vi "CollectImageSet (SubVI).vi"(0 "Session in":T1, 1 "Path to save collected images":path=path "E:/XYZstage+Camera_CollectedImages/12-17-2016/images", 3 "Stage position":refnum<vi>, 5 "Set of Coordinates to Process":dbl[][](array[numeric]), 8 "Current image":refnum<vi>, 9 "Axes Speeds [mm/s]":T4={"X Speed"=10.0, "Y Speed"=10.0, "Z Speed"=10.0}, 11 "error in":errorcluster, 13 "Moving":refnum<vi>) -> (4 "Session out":T1, 6 "Captured positions":dbl[][](array[numeric]), 10 "Image Array":T2[](array[plugin-control])=["remote image 0000000013A07714", "remote image 0000000013A076AC", "remote image 0000000013A0777C", "remote image 0000000013A077E4", "remote image 0000000013A0784C", "image_5", "image_6", "image_7", "image_8", "image_9", "image_10", "image_11", "image_12", "image_13", "image_14", "image_15", "image_16", "image_17", "image_18", "image_19", "image_20", "image_21", "image_22", "image_23", "image_24", "image_25", "image_26", "image_27", "image_28", "image_29", "image_30", "image_31", "image_32", "image_33", "image_34", "image_35", "image_36", "image_37", "image_38", "image_39", "image_40", "image_41", "image_42", "image_43", "image_44", "image_45", "image_46", "image_47", "image_48", "image_49", "image_50", "image_51", "image_52", "image_53", "image_54", "image_55", "image_56", "image_57", "image_58", "image_59", "image_60", "image_61", "image_62", "image_63", "image_64", "image_65", "image_66", "image_67", "image_68", "image_69", "image_70", "image_71", "image_72", "image_73", "image_74", "image_75", "image_76", "image_77", "image_78", "image_79"], 14 "Finished!":bool, 15 "error out":errorcluster)   [LabVIEW 2016]
uses:
  <vilib>/userdefined/High Color/IMAQdx.ctl
  <vilib>/vision/driver/NI_Vision_Acquisition_Software.lvlib
  <vilib>/vision/NI_Vision_Development_Module.lvlib
panel:
  out "Most recently collected image":T2(plugin-control)
  out "Image #":i32
  out "XYZ Stage Current Position":T3
  out "Moving":bool
  out "Object Location [mm]":T5
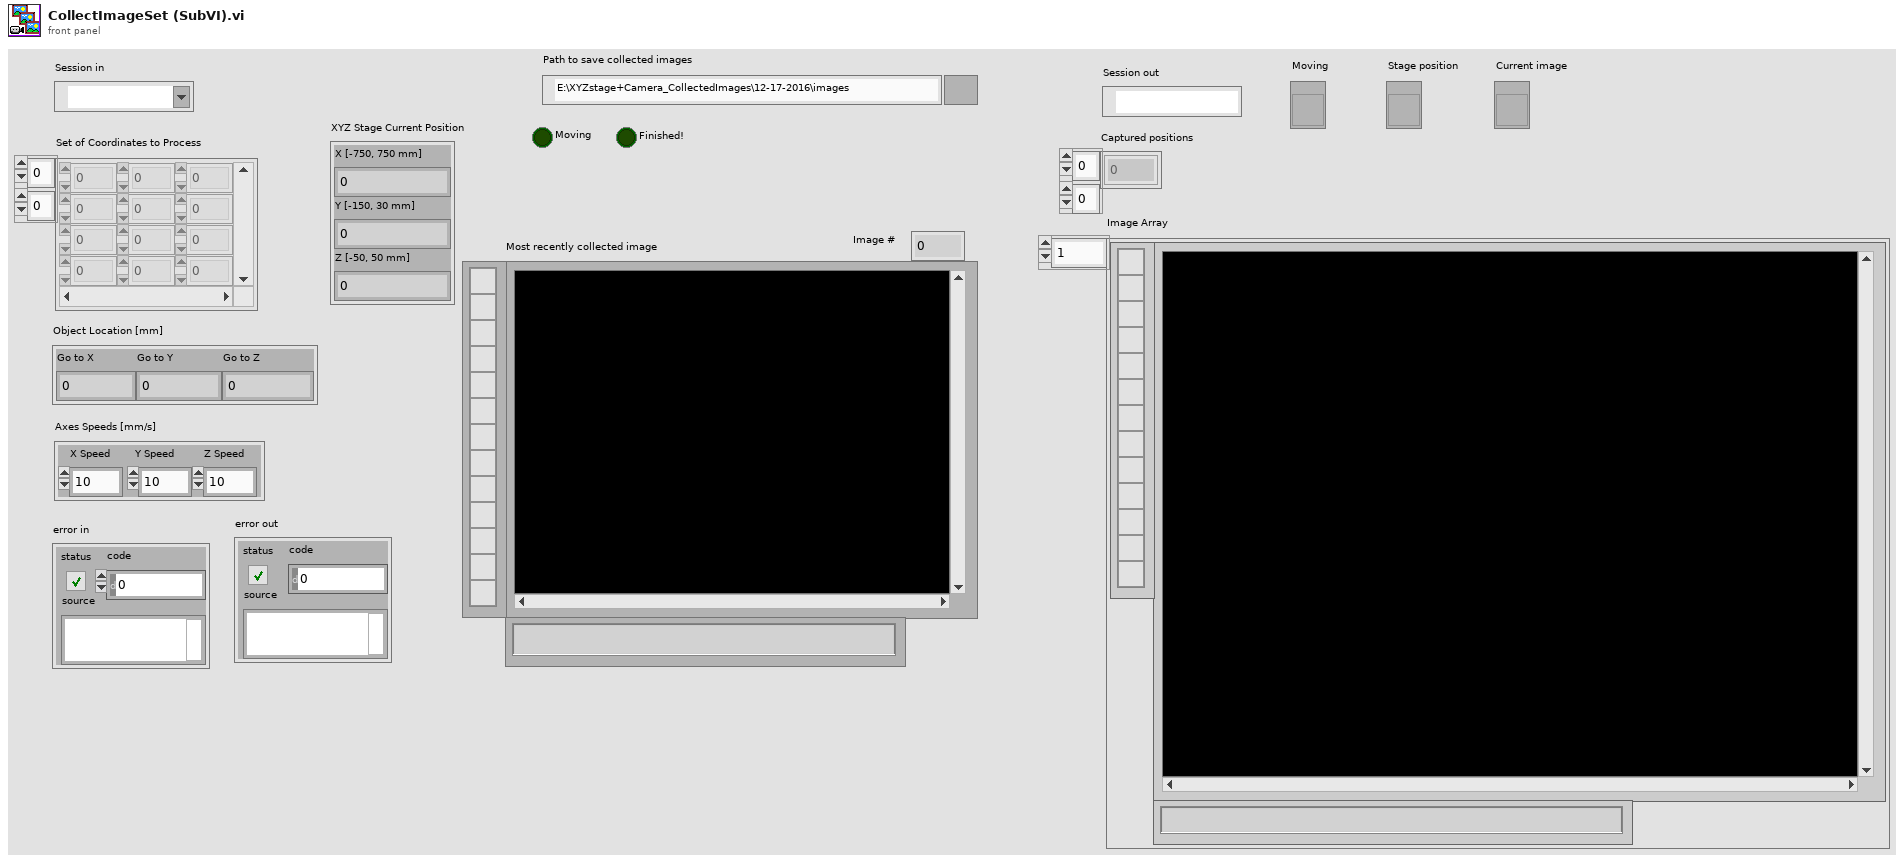
[diagram p1: front panel]
types:
  T1 = typedef "IMAQdx.ctl" = refnum<k21>
  T2 = typedef "IMAQ Image.ctl" = refnum<image>
  T3 = cluster{"X [-750, 750 mm]":dbl, "Y [-150, 30 mm]":dbl, "Z [-50, 50 mm]":dbl}
  T4 = cluster{"X Speed":dbl, "Y Speed":dbl, "Z Speed":dbl}
  T5 = cluster{"Go to X":dbl, "Go to Y":dbl, "Go to Z":dbl}
  T6 = cluster{"Set of Coordinates to Process[0]":dbl, "Set of Coordinates to Process[1]":dbl, "Set of Coordinates to Process[2]":dbl}
  T7 = typedef "Image Type" = u32
  T8 = cluster{"Final X":dbl, "Final Y":dbl, "Final Z":dbl}
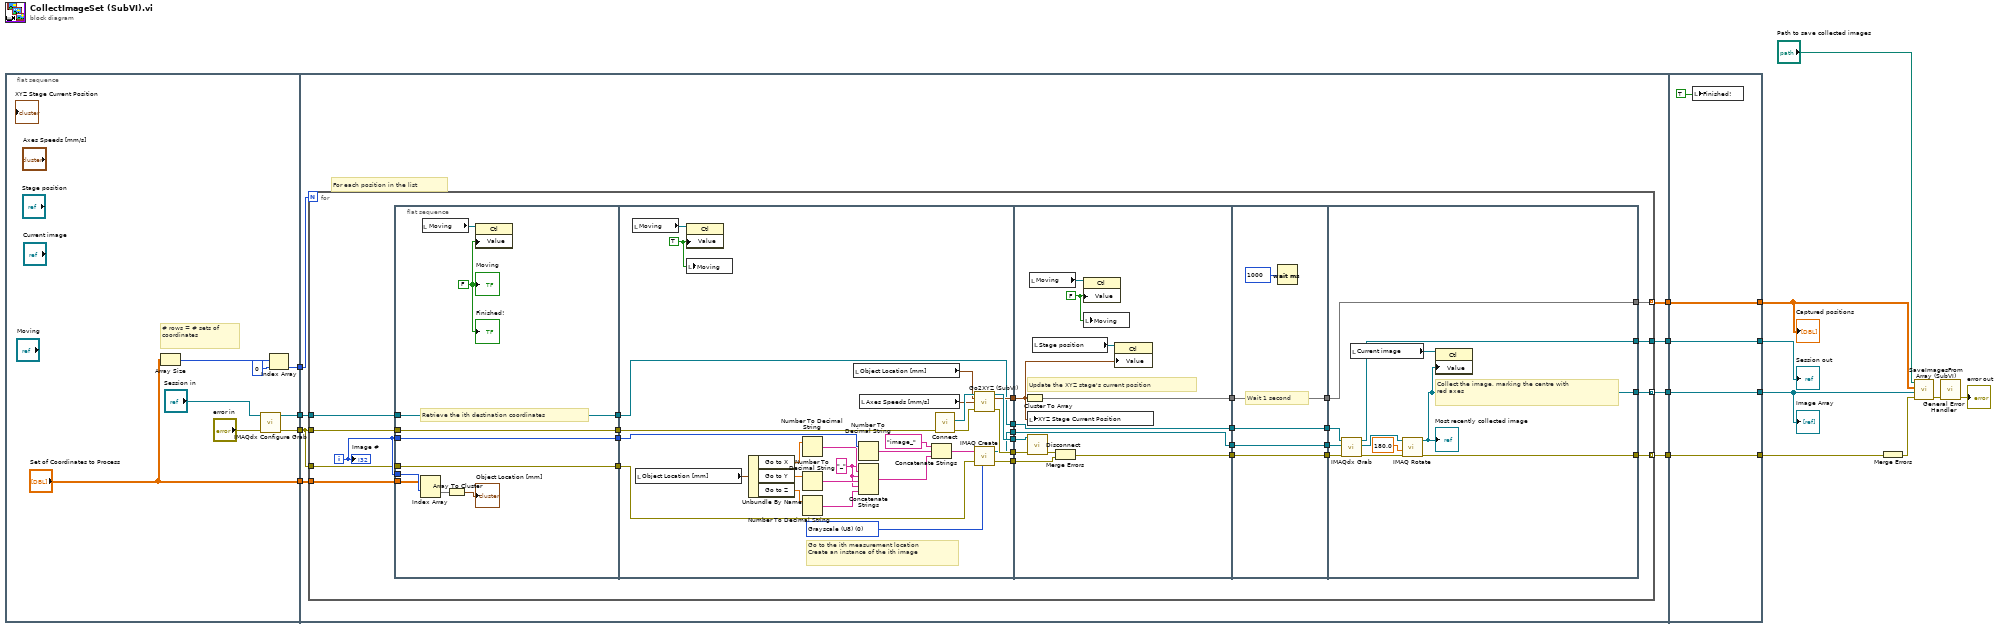
[diagram p0: block diagram]
diagram:
  n1 = flat-sequence {
    tunnel: [w18] -> w4
    tunnel: ["Set of Coordinates to Process"] -> w3
    tunnel: [w22] -> w2
    tunnel: [w21] -> w1
    tunnel: [w31] -> w16
    tunnel: [w30] -> w15
    tunnel: [w29] -> w14
    tunnel: [w28] -> w13
    tunnel: w4 -> [w32]
    tunnel: w3 -> [w27]
    tunnel: w2 -> [w26]
    tunnel: w1 -> [w25]
    tunnel: [w127] -> w12
    tunnel: [w128] -> w8
    tunnel: [w129] -> w11
    tunnel: [w130] -> w7
    tunnel: w16 -> [w130]
    tunnel: w15 -> [w129]
    tunnel: w14 -> [w128]
    tunnel: w13 -> [w127]
    frame #0 {
      # "# rows = # sets of\ncoordinates"
      n2 = Array Size(array="Set of Coordinates to Process") -> (size(s)=w20:i32[])
      n3 = call <vilib>:"IMAQdx Configure Grab.vi"("error in"="error in", "Session In"="Session in") -> ("error out"=w22:errorcluster, "Session Out"=w21:T1)  [unwired: 8 out]
      n4 = Index Array(array=w20, index=0) -> (element=w18:i32)
    }
    frame #1 {
      # "For each position in the list"
      n5 = for {
        N: w32 -> [_]
        tunnel: w25 -> [w47]
        tunnel: [w46] -> w31 mode=indexing
        tunnel: w26 -> [w44]
        tunnel: w26 -> [w42]
        tunnel: [w38] -> w30
        tunnel: [w37] -> w28 mode=indexing
        tunnel: [w34] -> w29 mode=indexing
        tunnel: w27 -> [w33]
        i -> [w55]
        n6 = flat-sequence {
          tunnel: w55 -> [w69]
          tunnel: w55 -> [w68]
          tunnel: [w68] -> w56
          tunnel: [w67] -> w48
          tunnel: w47 -> [w67]
          tunnel: [w66] -> w45
          tunnel: w44 -> [w66]
          tunnel: [w65] -> w43
          tunnel: w42 -> [w65]
          tunnel: w33 -> [w64]
          tunnel: [w94] -> w59
          tunnel: [w93] -> w58
          tunnel: [w92] -> w57
          tunnel: w56 -> [w87]
          tunnel: [w89] -> w52
          tunnel: [w88] -> w49
          tunnel: w48 -> [w88]
          tunnel: w45 -> [w85]
          tunnel: w43 -> [w81]
          tunnel: [w84] -> w39
          tunnel: w59 -> [w109]
          tunnel: w58 -> [w98]
          tunnel: w57 -> [w108]
          tunnel: [w107] -> w53
          tunnel: w52 -> [w107]
          tunnel: [w106] -> w50
          tunnel: w49 -> [w106]
          tunnel: [w103] -> w40
          tunnel: w39 -> [w104]
          tunnel: [w102] -> w36
          tunnel: [w113] -> w54
          tunnel: w53 -> [w113]
          tunnel: [w112] -> w51
          tunnel: w50 -> [w112]
          tunnel: [w111] -> w41
          tunnel: w40 -> [w111]
          tunnel: w36 -> [w110]
          tunnel: [w110] -> w35
          tunnel: w54 -> [w125]
          tunnel: w51 -> [w124]
          tunnel: [w115] -> w46
          tunnel: w41 -> [w121]
          tunnel: [w119] -> w38
          tunnel: [w117] -> w37
          tunnel: w35 -> [w118]
          tunnel: [w118] -> w34
          frame #0 {
            w60 = FALSE ("Finished!")
            # "Retrieve the ith destination coordinates"
            n7 = Index Array(array=w64, index (row)=w69) -> (element=w63:dbl[])  [unwired: 1 in]
            n8 = local read "Moving"() -> (w61:refnum<vi>)
            n9 = Array To Cluster(array=w63) -> (cluster=→"Object Location [mm]":T6)
            n10 = property class="Ctl"(reference=w61, "Value"=w60) -> ()  [unwired: 1 in, 2 out]
            "Finished!" <- w60
            "Moving" <- w60
          }
          frame #1 {
            w73 = "_" ("string")
            w70 = TRUE ("Moving")
            w97 = T7 0 items=["Grayscale (U8)", "Grayscale (I16)", "Grayscale (SGL)", "Complex (CSG)", "RGB (U32)", "HSL (U32)", "RGB (U64)", "Grayscale (U16)"] ("Image Type")
            # "Go to the ith measurement location\nCreate an instance of the ith image"
            n11 = local read "Moving"() -> (w71:refnum<vi>)
            n12 = local read "Object Location [mm]"() -> (w80:T5)
            n13 = property class="Ctl"(reference=w71, "Value"=w70) -> ()  [unwired: 1 in, 2 out]
            n14 = local write "Moving"(w70) -> ()
            n15 = Unbundle By Name(w80) -> ("Go to X"=w79:dbl, "Go to Y"=w78:dbl, "Go to Z"=w77:dbl)
            n16 = Number To Decimal String(number=w79) -> (decimal integer string=w76:string)  [unwired: 1 in]
            n17 = Number To Decimal String(number=w78) -> (decimal integer string=w75:string)  [unwired: 1 in]
            n18 = Number To Decimal String(number=w77) -> (decimal integer string=w74:string)  [unwired: 1 in]
            n19 = local read "Object Location [mm]"() -> (w82:T5)
            n20 = Number To Decimal String(number=w87) -> (decimal integer string=w86:string)  [unwired: 1 in]
            n21 = Concatenate Strings(w73, w76, w73, w75, w73, w74) -> (w72:string)
            n22 = local read "Axes Speeds [mm/s]"() -> (w83:T4)
            n23 = Concatenate Strings("image_" ("Image Name"), w86, w72) -> (w90:string)
            n24 = call "Connect.vi"("error in (no error)"=w85) -> ("error out"=w95:errorcluster, "controller"=w96:refnum<k24>)  [unwired: 9 in]
            n25 = call "Go2XYZ (SubVI).vi"(".NET Refnum in"=w96, "Go to Coordinates"=w82, "Axis Speeds"=w83, "error in (no error)"=w95) -> (".NET Refnum out"=w94:refnum<k24>, "Final Position"=w93:T8, "error out"=w92:errorcluster)  [unwired: 7 in, 2 out]
            n26 = call "IMAQ Create"("Image Name"=w90, "Image Type"=w97, "error in (no error)"=w81) -> ("New Image"=w89:T2, "error out"=w84:errorcluster)  [unwired: 1 in, 1 out]
          }
          frame #2 {
            w100 = FALSE ("Moving")
            # "Update the XYZ stage's current position"
            n27 = Cluster To Array(cluster=w98) -> (array=w102:dbl[])
            n28 = local write "XYZ Stage Current Position"(w98) -> ()
            n29 = call "Disconnect.vi"("error in (no error)"=w108, "controller"=w109) -> ("error out"=w105:errorcluster)  [unwired: 9 in]
            n30 = local read "Moving"() -> (w101:refnum<vi>)
            n31 = local read "Stage position"() -> (w99:refnum<vi>)
            n32 = Merge Errors(w105, w104) -> (w103:errorcluster)
            n33 = property class="Ctl"(reference=w101, "Value"=w100) -> ()  [unwired: 1 in, 2 out]
            n34 = local write "Moving"(w100) -> ()
            n35 = property class="Ctl"(reference=w99, "Value"=w98) -> ()  [unwired: 1 in, 2 out]
          }
          frame #3 {
            # "Wait 1 second"
            n36 = Wait (ms)(milliseconds to wait=u32 1000) -> ()  [unwired: 1 out]
          }
          frame #4 {
            # "Collect the image, marking the centre with \nred axes"
            n37 = call <vilib>:"IMAQdx Grab.vi"("error in"=w121, "Image In"=w125, "Session In"=w124) -> ("error out"=w120:errorcluster, "Image Out"=w123:T2, "Session Out"=w119:T1)  [unwired: 1 in, 5 out]
            n38 = local read "Current image"() -> (w116:refnum<vi>)
            n39 = call "IMAQ Rotate"("error in (no error)"=w120, "Angle (degrees)"=sgl 180.0, "Image Src"=w123) -> ("error out"=w117:errorcluster, "Image Dst Out"=w115:T2)  [unwired: 7 in]
            "Most recently collected image" <- w115
            n40 = property class="Ctl"(reference=w116, "Value"=w115) -> ()  [unwired: 1 in, 2 out]
          }
        }
        "Image #" <- w55
      }
    }
    frame #2 {
      n41 = local write "Finished!"(TRUE ("Finished!")) -> ()
    }
  }
  n42 = Merge Errors(w12) -> (w6:errorcluster)
  n43 = call "SaveImagesFromArray (SubVI).vi"("error in (no error)"=w6, "Array of Images"=w7, "XY Camera Coordinates"=w8, "Path to save collected images"="Path to save collected images") -> ("error out"=w5:errorcluster)  [unwired: 7 in]
  n44 = call <vilib>:"General Error Handler.vi"("error in (no error)"=w5) -> ("error out"=→"error out":errorcluster)  [unwired: 2 in, 12 out]
  "Image Array" <- w7
  "Captured positions" <- w8
  "Session out" <- w11
